vi "Format String.vi"(8 "error in (no error)":errorcluster, 10 "String In":string, 11 "Fluke Calibrator in":refnum<class "Fluke Calibrator.lvclass">) -> (0 "error out":errorcluster, 2 "Number out":dbl, 3 "Fluke Calibrator out":refnum<class "Fluke Calibrator.lvclass">)   [LabVIEW 2012, in "Fluke Calibrator.lvclass"]
uses:
  Fluke Calibrator.lvclass
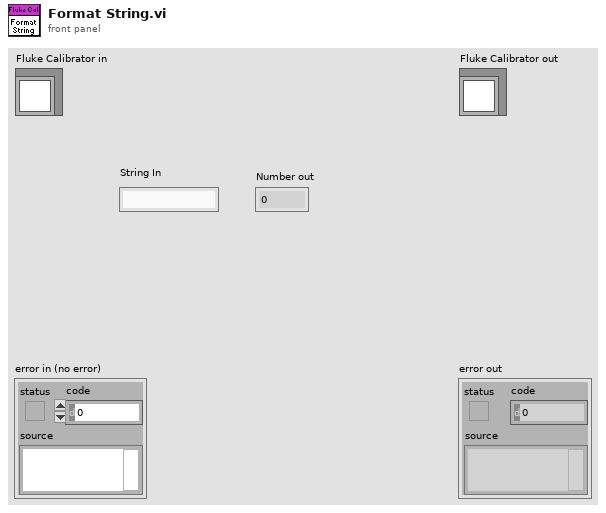
[diagram p1: front panel]
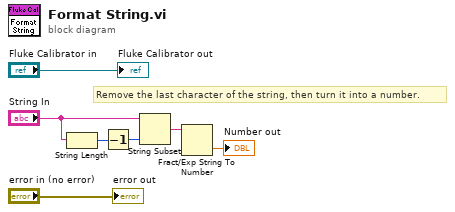
[diagram p0: block diagram]
diagram:
  # "Remove the last character of the string, then turn it into a number."
  n1 = String Length(string="String In") -> (length=w7:i32)
  n2 = Decrement(x=w7) -> (x-1=w6:i32)
  n3 = String Subset(string="String In", length (rest)=w6) -> (substring=w5:string)  [unwired: 1 in]
  n4 = Fract/Exp String To Number(string=w5) -> (number=→"Number out":dbl)  [unwired: 3 in, 1 out]
  "error out" <- "error in (no error)"
  "Fluke Calibrator out" <- "Fluke Calibrator in"
